vi "Go_to_State3.vi"(8 "error in (no error)":errorcluster, 11 "Demo_States in":refnum<class "Demo_States.lvclass">) -> (0 "error out":errorcluster, 3 "State out":refnum<class "State Actor.lvclass">)   [LabVIEW 2025, in "Demo_States.lvlib" / "Demo_States.lvclass"]
uses:
  Demo_States.lvclass
  <vilib>/ni/Actors/State Actor/State Actor/State Actor.lvclass
  State3/State3.lvclass
  demo Messages/Log State Msg/Log State Msg.lvclass
  <vilib>/ActorFramework/Actor/Actor.lvclass
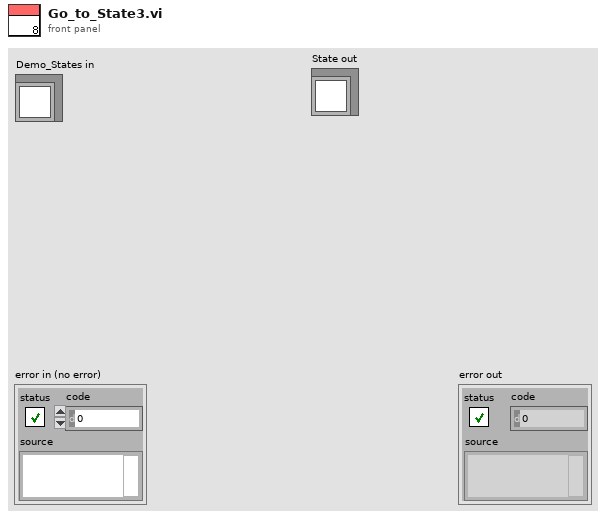
[diagram p1: front panel]
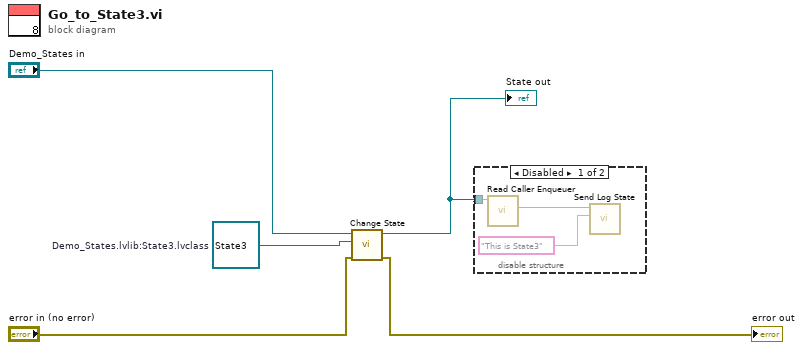
[diagram p0: block diagram]
diagram:
  w2 = refnum<class "State3.lvclass"> refnum  # Demo_States.lvlib:State3.lvclass
  n1 = call <vilib>:"Change State.vi"("error in (no error)"="error in (no error)", "New State in"=w2, "State in"="Demo_States in") -> ("error out"=→"error out":errorcluster, "State out"=w1:refnum<class "State Actor.lvclass">)  [unwired: 7 in]
  "State out" <- w1
  n2 = disable-structure shown="Disabled" {
    disable-tunnel: w1 -> [w8 _]
    frame Disabled {
      n3 = call <vilib>:"Read Caller Enqueuer.vi"("Actor"=w8) -> ("Caller Enqueuer"=w7:refnum<class "Message Enqueuer.lvclass">)  [unwired: 10 in]
      n4 = call "Send Log State.vi"("State"="This is State3", "Message Enqueuer"=w7) -> ()  [unwired: 8 in, 2 out]
    }
    frame Enabled {
    }
  }
